vi "HAL sim (SubVI).vi"(10 "stop in":bool, 11 "Notifier in":refnum<notifier>) -> ()   [LabVIEW 2014]
uses:
  MATH/MathLoop/TypeDefs/ParsedExpression.ctl
  MATH/MathLoop/TypeDefs/typeMed.ctl
  MATH/MathLoop/TypeDefs/Conf. Gral.ctl
  MATH/MathLoop/MathLoop.lvlib
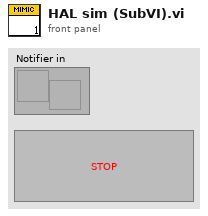
[diagram p1: front panel]
types:
  T1 = typedef "MathLoop.lvlib/Conf. Gral.ctl" = cluster{"Engranometro":cluster{"Cant. Dientes x pieza":i32, "Nro. Dientes (Frp)":i32, "Armonicas":i32}}
  T2 = cluster{"Kcte":sgl[], "Dcte":sgl[], "Aux":sgl[][], "Transductores":sgl[][]}
  T3 = typedef "MathLoop.lvlib/ParsedExpression.ctl" = cluster{"RPN ":string[], "Constantes":sgl[], "Variables":string[], "Formula":string, "Tipo de Med":T4, "Med?":bool, "Descripción":string, "Nominal":sgl, "Tol Sup":sgl, "Pre TS":sgl, "Pre TI":sgl, "Tol Inf":sgl}
  T4 = typedef "MathLoop.lvlib/typeMed.ctl" = string
  T5 = cluster{"Variable Data Out":cluster{"Kcte":sgl[], "Dcte":sgl[], "Aux":sgl[][], "Transductores":sgl[][]}, "Array":sgl[], T3[], "Array Med":sgl[][], "Conf. General":T1}
  T6 = cluster{"RPN ":string[], "Constantes":sgl[], "Variables":string[], "Formula":string, "Tipo de Med":string, "Med?":bool, "Descripción":string, "Nominal":sgl, "Tol Sup":sgl, "Pre TS":sgl, "Pre TI":sgl, "Tol Inf":sgl}
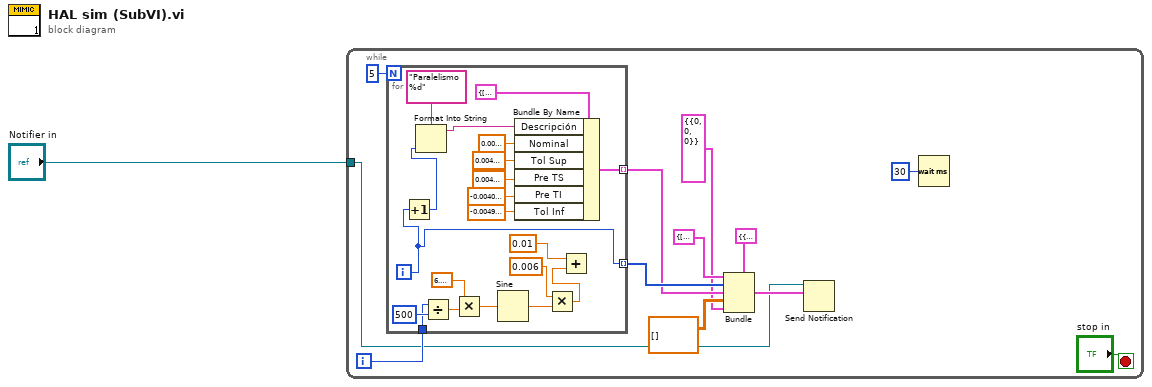
[diagram p0: block diagram]
diagram:
  n1 = while {
    tunnel: "Notifier in" -> [w3]
    i -> [w8]
    stop <- "stop in" stop-if-true
    n2 = for {
      N: 5 -> [_]
      tunnel: [w14] -> w10 mode=indexing
      tunnel: w8 -> [w18]
      tunnel: [w16] -> w7 mode=indexing
      i -> [w14]
      n3 = Increment(x=w14) -> (x+1=w15:i32)
      n4 = Format Into String(format string="Paralelismo %d", w15) -> (resulting string=w17:string)  [unwired: 2 in, 1 out]
      n5 = Divide(x=w18, y=500) -> (x/y=w26:dbl)
      n6 = Multiply(x=6.283185307179586, y=w26) -> (x*y=w24:dbl)
      n7 = Sine(x=w24) -> (sin(x)=w23:dbl)
      n8 = Bundle By Name(cluster=T6 {"RPN "=[], "Constantes"=[], "Variables"=[], "Formula"="", "Tipo de Med"="", "Med?"=FALSE, "Descripción"="", "Nominal"=0.0, "Tol Sup"=0.0, "Pre TS"=0.0, "Pre TI"=0.0, "Tol Inf"=0.0} ("Parsed Expression Out"), "Descripción"=w17, "Nominal"=sgl 0.01, "Tol Sup"=sgl 0.005, "Pre TS"=sgl 0.004, "Pre TI"=sgl -0.004, "Tol Inf"=sgl -0.005) -> (w16:T6)
      n9 = Multiply(x=0.006 ("y"), y=w23) -> (x*y=w21:dbl)
      n10 = Add(x=0.01, y=w21) -> ()  [unwired: 1 out]
    }
    n11 = Bundle(cluster=T5 {"Variable Data Out"={"Kcte"=[], "Dcte"=[], "Aux"=[], "Transductores"=[]}, "Array"=[], [], "Array Med"=[], "Conf. General"={"Engranometro"={"Cant. Dientes x pieza"=0, "Nro. Dientes (Frp)"=0, "Armonicas"=0}}} ("output cluster"), "Variable Data Out"=T2 {"Kcte"=[], "Dcte"=[], "Aux"=[], "Transductores"=[]}, "Array"=w10, w7, "Array Med"=sgl[][] [], "Conf. General"=T1 {"Engranometro"={"Cant. Dientes x pieza"=0, "Nro. Dientes (Frp)"=0, "Armonicas"=0}}) -> (w12:T5)
    n12 = Send Notification(notification=w12, notifier=w3) -> ()  [unwired: 1 in, 2 out]
    n13 = Wait (ms)(milliseconds to wait=u32 30) -> ()  [unwired: 1 out]
  }
